vi "Build Result Channel Name from Wfm System Definition Path.vi"(8 "error in (no error)":errorcluster, 11 "Channel Path":string="Targets/Controller/Hardware/Chassis/DAQ/DAQ1/Analog Input/AI0") -> (0 "error out":errorcluster, 3 "delimited string":string)   [LabVIEW 2015, in "Waveform-Processing-Custom-Device System Explorer.lvlib"]
uses:
  Waveform-Processing-Custom-Device System Explorer.lvlib
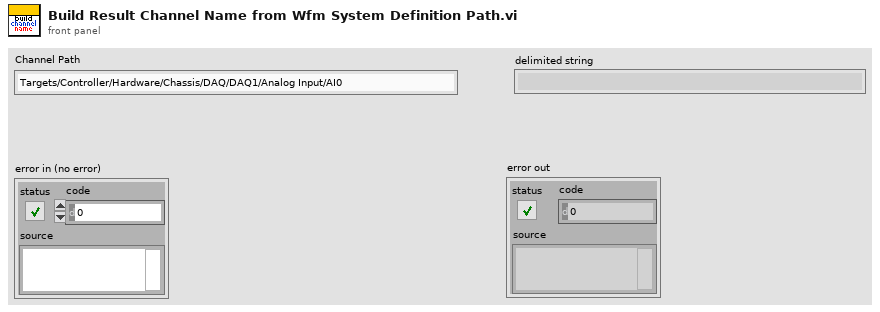
[diagram p1: front panel]
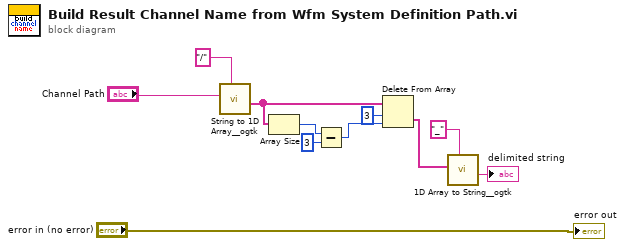
[diagram p0: block diagram]
diagram:
  n1 = call <userlib>:"String to 1D Array__ogtk.vi"("delimiter (Tab)"="/", "string"="Channel Path") -> ("Array of Strings"=w10:string[])  [unwired: 9 in]
  n2 = Array Size(array=w10) -> (size(s)=w9:i32)
  n3 = Subtract(x=w9, y=3) -> (x-y=w7:i32)
  n4 = Delete From Array(array=w10, length=3, index=w7) -> (deleted portion=w5:string[])  [unwired: 1 out]
  n5 = call <userlib>:"1D Array to String__ogtk.vi"("delimiter (Tab)"="_", "Array of Strings"=w5) -> ("delimited string"=→"delimited string":string)  [unwired: 9 in]
  "error out" <- "error in (no error)"
